vi "play_AFMss_fp_distEst_deltaUk.vi"() -> ()   [LabVIEW 2017]
uses:
  <vilib>/Analysis/Matrix/Datatypes/RealMatrix.ctl
  fpga_fp_interface_lib/fpga_interface_types/boolean_indicators.ctl
  controls/ControlParams.ctl
  controls/controlParams_tracktraj.ctl
  <vilib>/userdefined/High Color/nirio_resource_hc.ctl
  <vilib>/Utility/error.llb/DialogType.ctl
  <vilib>/Utility/file.llb/Read From Spreadsheet File (DBL).vi
  <vilib>/FPGAPlugInAG/cRIO-9082/niLvFpga_Open_cRIO-9082.vi
  <vilib>/rvi/interface/common/dynamic/niFpgaDynamicAddResources.vi
  <vilib>/FPGAPlugInAG/Dynamic/niLvFpga_Reset_Dynamic.vi
  <vilib>/rvi/interface/common/niFpgaWaitOnOcc.vi
  <vilib>/Utility/error.llb/Error Cluster From Error Code.vi
  <vilib>/rvi/errors/niLvFpgaAdjustHostInterfaceError.vi
  <vilib>/FPGAPlugInAG/Dynamic/niLvFpga_Run_Dynamic.vi
  <vilib>/Utility/file.llb/Write To Spreadsheet File (DBL).vi
  <vilib>/FPGAPlugInAG/Dynamic/niLvFpga_Close_Dynamic.vi
  <vilib>/rvi/interface/nirviOpenFPGA/nirviOpenFPGA.xnode
  FPGA Bitfiles/XYpeizocontrol_AFMss_control_trajTrack_deltaU_distEst.lvbitx
  <vilib>/rvi/interface/nirviMethod/nirviMethod.xnode
  <vilib>/rvi/interface/nirviReadWriteControl/nirviReadWriteControl.xnode
  <vilib>/rvi/interface/nirviCloseFPGA/nirviCloseFPGA.xnode
  <vilib>/FPGAPlugInAG/Dynamic/niLvFpga_ConfigureFifo_Dynamic.vi
  <vilib>/rvi/errors/niLvFpgaMergeErrorWithErrorCode.vi
  NiFpgaLv.dll
  <vilib>/rvi/interface/Simulation/niFpgaSimulationCallBeginRW.vi
  labview/utils_lib/utils.lvlib
  <vilib>/FPGAPlugInAG/Dynamic/niLvFpga_WriteFifo_Dynamic.vi
  <vilib>/Analysis/Matrix/NI_Matrix.lvlib
panel:
  out "output cluster":T1={"umax"=3.0, "y_ref(k)"=0.0, "Ki"=0.0, "y(k) (from plant)"=0.0, "ND"=0, "NS"=0, "u_Kx_ref(k)"=0.0, "du_max"=3.0, "NS_obs"=0, "NS_control"=0} {"du_max" format="%#_13g"; "u_Kx_ref(k)" format="%#_13g"; "Ki" format="%#_13g"; "y_ref(k)" format="%#_13g"; "umax" format="%#_13g"}
  out "controlParams":T2={"NS"=7, "ND"=10, "Nbar"=1.253469179440319, "Ki"=0.125346917944, "ref"=0.125346917944} {"ref" format="%#_13g"; "Ki" format="%#_13g"; "Nbar" format="%#_13g"}
  out "x+y":i32
  in  "du_max":dbl=1.0 format="%#_13g"
  out "uk_fifo_size":i32[](array[numeric])
  out "yk_fifo_size":i32[](array[numeric])
  out "boolean  indicators":T3
  out "Unstable Traj":bool
  in  "ABORT":bool
  in  "N_hyst":i32
  in  "w-s":T4
  in  "r_s":T4
  in  "TF Order":i32
  in  "den":T4
  in  "num":T4
  out "elements left":i32=1
  in  "control_data_path":path=path "Z:/mpc-journal/step-exps/exp01Controls.csv"
  out "Actual Depth":u32
  in  "reference traj path":path=path "Z:/mpc-journal/step-exps/ref_traj_track.csv"
  in  "outputData BOTH":path=path "Z:/mpc-journal/step-exps/exp01outputBOTH.csv"
  in  "SettleTicks":i32=10
  out "u iter":i32
  out "Elements Remaining":u32
  out "Control Loop Done":bool
  out "yk":sgl
  out "UK TO":bool
  out "YK TO":bool
  in  "Iters":i32=25
  in  "Cont Run (F)":bool=TRUE
  in  "ymax":dbl=4.0 format="%#_13g"
  in  "umax":dbl=1.0 format="%#_13g"
  in  "TsTicks":i32=1600
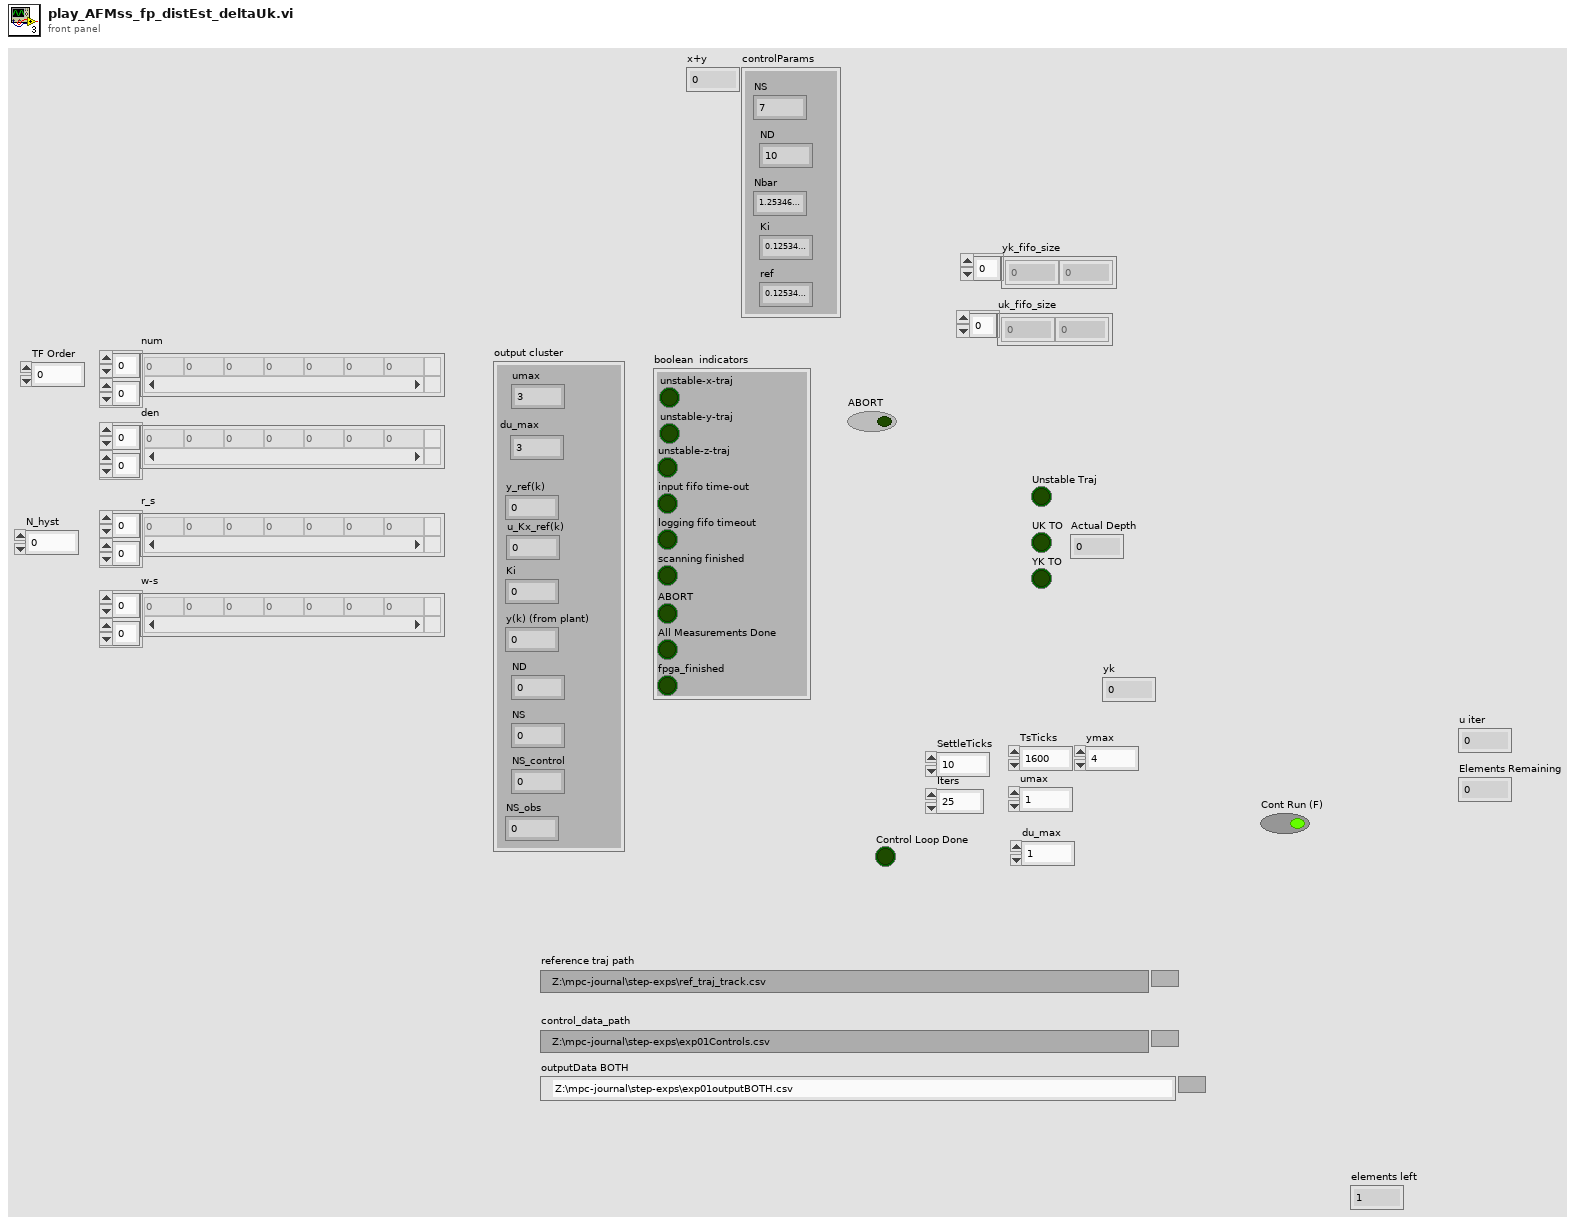
[diagram p1: front panel]
types:
  T1 = typedef "controlParams_tracktraj.ctl" = cluster{"umax":sgl, "y_ref(k)":sgl, "Ki":sgl, "y(k) (from plant)":sgl, "ND":i16, "NS":i16, "u_Kx_ref(k)":sgl, "du_max":sgl, "NS_obs":i16, "NS_control":i16}
  T2 = typedef "ControlParams.ctl" = cluster{"NS":i32, "ND":i32, "Nbar":dbl, "Ki":dbl, "ref":dbl}
  T3 = typedef "boolean_indicators.ctl" = cluster{"unstable-z-traj":bool, "input fifo time-out":bool, "logging fifo timeout":bool, "scanning finished":bool, "unstable-x-traj":bool, "unstable-y-traj":bool, "ABORT":bool, "All Measurements Done":bool, "fpga_finished":bool}
  T4 = typedef "NI_Matrix.lvlib/RealMatrix.ctl" = dbl[][]
  T5 = typedef "nirio_resource_hc.ctl" = tag
  T6 = typedef "DialogType.ctl" = u16
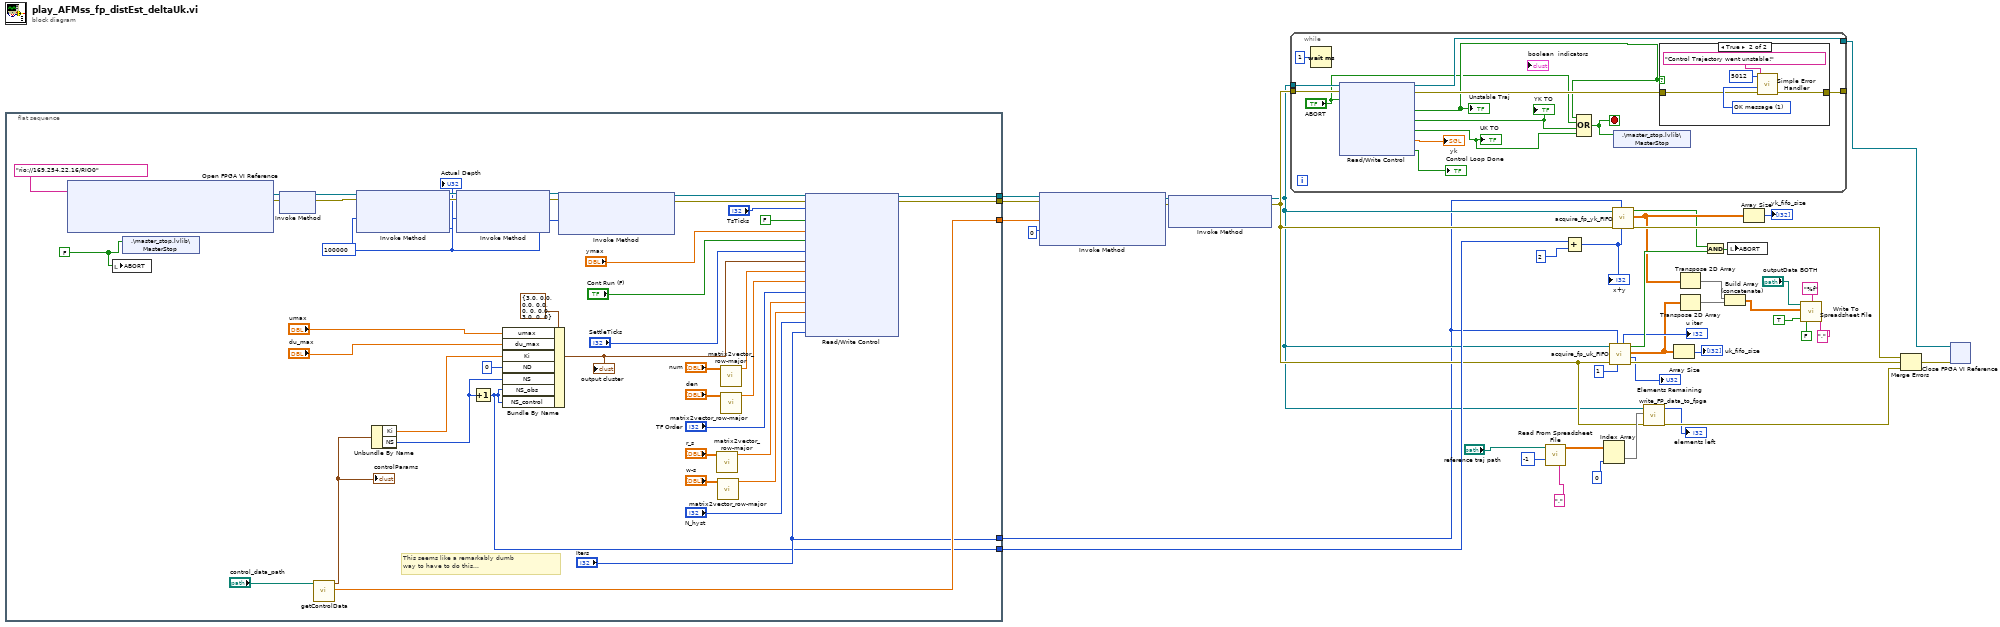
[diagram p0: block diagram]
diagram:
  n1 = flat-sequence {
    tunnel: [w64] -> w23
    tunnel: [w63] -> w21
    tunnel: [w62] -> w20
    tunnel: [w43] -> w8
    tunnel: ["Iters"] -> w2
    frame #0 {
      w49 = FALSE
      w72 = 100000
      # "This seems like a remarkably dumb\nway to have to do this..."
      n2 = xnode "Open FPGA VI Reference"("resource name"=T5 "rio://169.254.22.16/RIO0") -> ("FPGA VI Reference Out"=w70:refnum<k20>, "error out"=w69:errorcluster)  [unwired: 1 in]
      n3 = local write "ABORT"(w49) -> ()
      n4 = shared-variable ".\\master_stop.lvlib\\MasterStop"(w49) -> ()  [unwired: 1 in, 1 out]
      n5 = xnode "Invoke Method"("FPGA VI Reference In"=w70, "error in"=w69) -> ("FPGA VI Reference Out"=w79:refnum<k20>, "error out"=w78:errorcluster)
      n6 = call "getControlData.vi"("system matricec path"="control_data_path") -> ("AllMatrix"=w64:dbl[], "controlParams"=w71:T2)  [unwired: 9 in]
      "controlParams" <- w71
      n7 = xnode "Invoke Method"("FPGA VI Reference In"=w79, "error in"=w78, "Requested Depth"=w72) -> ("FPGA VI Reference Out"=w85:refnum<k20>, "error out"=w84:errorcluster, "Actual Depth"=→"Actual Depth":u32)
      n8 = Unbundle By Name(w71) -> ("Ki"=w61:dbl, "NS"=w44:i32)
      n9 = xnode "Invoke Method"("FPGA VI Reference In"=w85, "error in"=w84, "Requested Depth"=w72) -> ("FPGA VI Reference Out"=w76:refnum<k20>, "error out"=w75:errorcluster)  [unwired: 1 out]
      n10 = Increment(x=w44) -> (x+1=w43:i32)
      n11 = Bundle By Name(cluster=T1 {"umax"=3.0, "y_ref(k)"=0.0, "Ki"=0.0, "y(k) (from plant)"=0.0, "ND"=0, "NS"=0, "u_Kx_ref(k)"=0.0, "du_max"=3.0, "NS_obs"=0, "NS_control"=0} ("Cluster"), "umax"="umax", "du_max"="du_max", "Ki"=w61, "ND"=i16 0, "NS"=w44, "NS_obs"=w43, "NS_control"=w43) -> (w68:T1)
      "output cluster" <- w68
      n12 = xnode "Invoke Method"("FPGA VI Reference In"=w76, "error in"=w75, "Requested Depth"=w72) -> ("FPGA VI Reference Out"=w74:refnum<k20>, "error out"=w73:errorcluster)  [unwired: 1 out]
      n13 = call "matrix2vector_row-major.vi"("Matrix"="r_s") -> ("vector"=w53:dbl[])  [unwired: 10 in]
      n14 = call "matrix2vector_row-major.vi"("Matrix"="w-s") -> ("vector"=w52:dbl[])  [unwired: 10 in]
      n15 = call "matrix2vector_row-major.vi"("Matrix"="num") -> ("vector"=w60:dbl[])  [unwired: 10 in]
      n16 = call "matrix2vector_row-major.vi"("Matrix"="den") -> ("vector"=w57:dbl[])  [unwired: 10 in]
      n17 = xnode "Read/Write Control"("FPGA VI Reference In"=w74, "error in"=w73, "TsTicks"="TsTicks", "Abort"=FALSE, "ymax"="ymax", "False  = cont run"="Cont Run (F)", "Settle Ticks"="SettleTicks", "Cluster"=w68, "Num"=w60, "Den"=w57, "TF Order"="TF Order", "r_s"=w53, "w_s"=w52, "N_hyst"="N_hyst", "iters"="Iters") -> ("FPGA VI Reference Out"=w62:refnum<k20>, "error out"=w63:errorcluster)
    }
  }
  n18 = xnode "Invoke Method"("FPGA VI Reference In"=w20, "error in"=w21, "Data"=w23, "Timeout (ms)"=0) -> ("FPGA VI Reference Out"=w25:refnum<k20>, "error out"=w24:errorcluster)  [unwired: 1 out]
  n19 = xnode "Invoke Method"("FPGA VI Reference In"=w25, "error in"=w24) -> ("FPGA VI Reference Out"=w5:refnum<k20>, "error out"=w7:errorcluster)  [unwired: 1 in]
  n20 = while {
    tunnel: w5 -> [w97]
    tunnel: w7 -> [w96]
    tunnel: [w94] -> _
    tunnel: [w91] -> w15
    stop <- w88 stop-if-true
    n21 = Wait (ms)(milliseconds to wait=u32 1) -> ()  [unwired: 1 out]
    n22 = xnode "Read/Write Control"("FPGA VI Reference In"=w97, "error in"=w96, "Abort"="ABORT") -> ("FPGA VI Reference Out"=w91:refnum<k20>, "error out"=w95:errorcluster, "Unstable Traj"=w87:bool, "YK TO"=w90:bool, "UK TO"=w89:bool, "yk"=→"yk":sgl, "Loop Done"=→"Control Loop Done":bool)
    "YK TO" <- w90
    "UK TO" <- w89
    "Unstable Traj" <- w87
    n23 = Compound Arithmetic op=OR(w87, "ABORT", w90, w89) -> (w88:bool)
    n24 = shared-variable ".\\master_stop.lvlib\\MasterStop"(w88) -> ()  [unwired: 1 in, 1 out]
    n25 = case shown="True" w87 {
      tunnel: w95 -> [w99 w101]
      tunnel: [w99 w100] -> w94
      frame False {
      }
      frame True {
        w104 = T6 1 items=["no dialog", "OK message", "continue or stop message", "OK message + warnings", "continue/stop + warnings"] ("type of dialog (OK msg:1)")
        n26 = call <vilib>:"Simple Error Handler.vi"("error code (no error:0)"=5012, "error source (\" \")"="Control Trajectory went unstable!" ("error source (\" \")"), "type of dialog (OK msg:1)"=w104, "error in (no error)"=w101) -> ("error out"=w100:errorcluster)  [unwired: 1 in, 4 out]
      }
    }
  }
  n27 = call-poly <vilib>:"Read From Spreadsheet File.vi"("delimiter (\\t)"=",", "number of rows (all:-1)"=-1, "file path (dialog if empty)"="reference traj path") -> ("all rows"=w31:dbl[][])  [unwired: 4 in, 4 out]
  n28 = Add(x=w8, y=2) -> (x+y=w3:i32)
  "x+y" <- w3
  n29 = Index Array(array=w31, index (col)=0 ("dimension size")) -> (element=w30:dbl[])  [unwired: 1 in]
  n30 = call "acquire_fp_uk_FIFO.vi"("numChannels"=i16 1, "Iters"=w2, "error in (no error)"=w7, "FPGA Interface"=w5) -> ("error out"=w28:errorcluster, "Elements Remaining"=→"Elements Remaining":u32, "2D Data Out"=w11:dbl[][], "acquisition done"=w19:bool, "u iter"=→"u iter":i32)  [unwired: 3 in]
  n31 = call "acquire_fp_yk_FIFO.vi"("numChannels"=w3, "Iters"=w2, "error in (no error)"=w7, "FPGA Interface"=w5) -> ("error out"=w6:errorcluster, "2D Data Out"=w4:dbl[][], "acquisition done"=w1:bool)  [unwired: 3 in, 2 out]
  n32 = call "write_FP_data_to_fpga.vi"("error in"=w7, "all rows"=w30, "FPGA Interface"=w5) -> ("error out"=w27:errorcluster, "elements left"=→"elements left":i32)  [unwired: 7 in]
  n33 = Array Size(array=w11) -> (size(s)=→"uk_fifo_size":i32[])
  n34 = Transpose 2D Array(2D array=w4) -> (transposed array=w42:dbl[][])
  n35 = Transpose 2D Array(2D array=w11) -> (transposed array=w41:dbl[][])
  n36 = And(x=w1, y=w19) -> (x .and. y?=w18:bool)
  n37 = Build Array (concatenate)(w42, w41) -> (w9:dbl[][])
  n38 = local write "ABORT"(w18) -> ()
  n39 = Array Size(array=w4) -> (size(s)=→"yk_fifo_size":i32[])
  n40 = call-poly <vilib>:"Write To Spreadsheet File.vi"("delimiter (\\t)"=",", "transpose? (no:F)"=TRUE, "format (%.3f)"="%f", "append to file? (new file:F)"=FALSE, "2D data"=w9, "file path (dialog if empty)"="outputData BOTH") -> ()  [unwired: 2 in, 1 out]
  n41 = Merge Errors(w6, w28, w27) -> (w29:errorcluster)
  n42 = xnode "Close FPGA VI Reference"("FPGA VI Reference In"=w15, "error in"=w29) -> ()  [unwired: 1 out]
